vi "alignHorizontalCentersWith.vi"(6 "useControlBodyOnly":bool, 8 "error in (no error)":errorcluster, 10 "anchorObject":refnum<vi>, 11 "movingObject":refnum<vi>) -> (0 "error out":errorcluster, 2 "anchorObject(dup)":refnum<vi>, 3 "movingObject(dup)":refnum<vi>)   [LabVIEW 2023, in "TLC_Geometry.lvlib"]
doc: "Aligns the horizontal center of the moving object with the horizontal center of the anchor control.\n\nOnly the X position of the item is modified.\nThe Y position is preserved."
uses:
  TLC_Geometry.lvlib
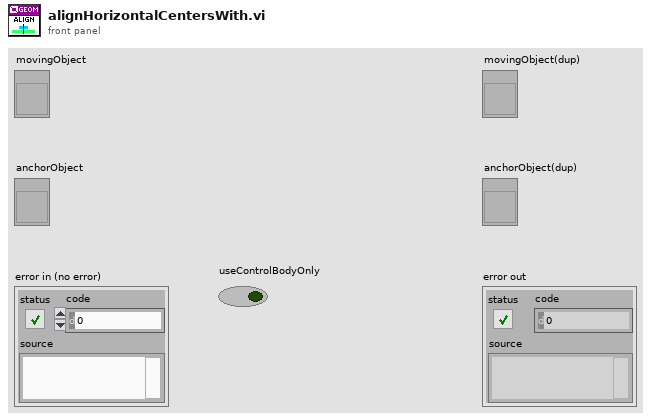
[diagram p1: front panel]
types:
  T1 = cluster{"left":i32, "top":i32, "right":i32, "bottom":i32}
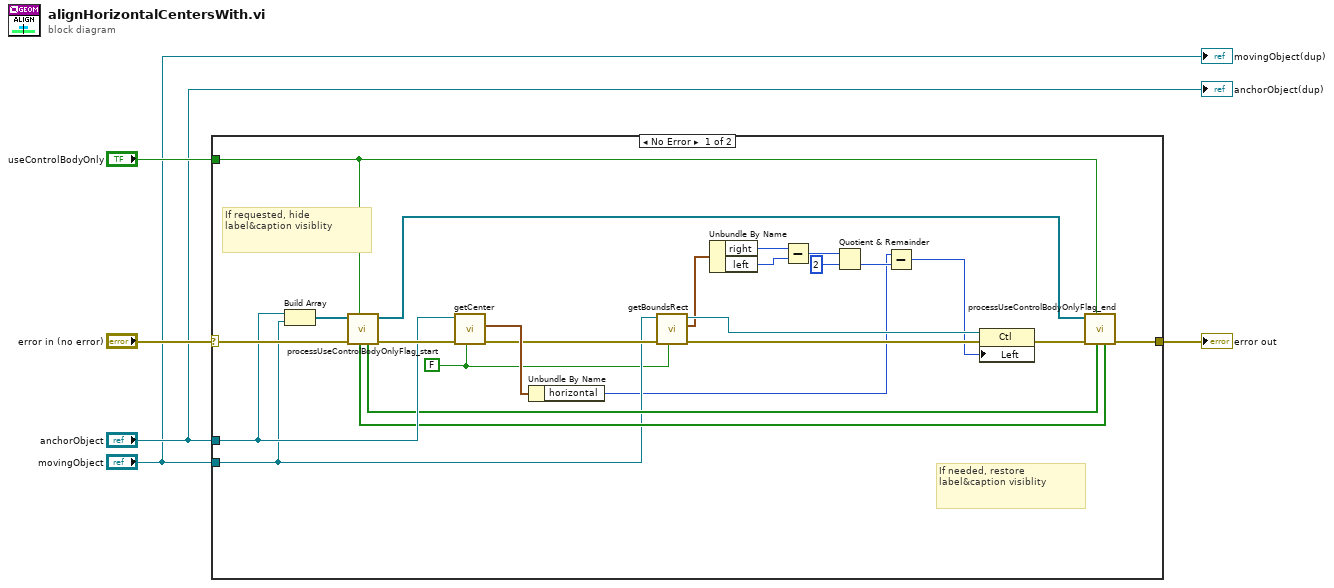
[diagram p0: block diagram]
diagram:
  n1 = case shown="No Error" "error in (no error)" {
    selector: "error in (no error)" -> [w29 w30]
    tunnel: [w26 w30] -> w5
    tunnel: "anchorObject" -> [w24 _]
    tunnel: "useControlBodyOnly" -> [w21 _]
    tunnel: "movingObject" -> [w11 _]
    frame No Error {
      w9 = FALSE ("ignoreCaption&Labels")
      # "If needed, restore label&caption visiblity"
      # "If requested, hide label&caption visiblity"
      n2 = Build Array(w24, w11) -> (w28:refnum<vi>[])
      n3 = call "processUseControlBodyOnlyFlag_start.vi"("useControlBodyOnly"=w21, "error in (no error)"=w29, "refList"=w28) -> ("error out"=w25:errorcluster, "refList(dup)"=w27:refnum<vi>[], "LabelVisibilityList"=w20:bool[], "captionVisibilityList"=w19:bool[])  [unwired: 5 in]
      n4 = call "getCenter.vi"("useControlBodyOnly"=w9, "error in (no error)"=w25, "ref"=w24) -> ("error out"=w14:errorcluster, "center"=w23:cluster{"horizontal":i32, "vertical":i32})  [unwired: 6 in, 1 out]
      n5 = Unbundle By Name(w23) -> ("horizontal"=w7:i32)
      n6 = call "getBoundsRect.vi"("useControlBodyOnly"=w9, "error in (no error)"=w14, "ref"=w11) -> ("error out"=w13:errorcluster, "rect"=w10:T1, "ref(dup)"=w12:refnum<vi>)  [unwired: 6 in]
      n7 = Unbundle By Name(w10) -> ("right"=w18:i32, "left"=w17:i32)
      n8 = Subtract(x=w18, y=w17) -> (x-y=w15:i32)
      n9 = Quotient & Remainder(x=w15, y=2) -> (floor(x/y)=w16:i32)  [unwired: 1 out]
      n10 = Subtract(x=w7, y=w16) -> (x-y=w6:i32)
      n11 = property class="Ctl"(reference=w12, error in=w13, "Left"=w6) -> (error out=w22:errorcluster)  [unwired: 1 out]
      n12 = call "processUseControlBodyOnlyFlag_end.vi"("captionVisibilityList"=w19, "LabelVisibilityList"=w20, "useControlBodyOnly"=w21, "error in (no error)"=w22, "refList"=w27) -> ("error out"=w26:errorcluster)  [unwired: 5 in, 1 out]
    }
    frame Error {
    }
  }
  "error out" <- w5
  "movingObject(dup)" <- "movingObject"
  "anchorObject(dup)" <- "anchorObject"
